vi "Populate_Do.vi"(8 "error in (no error)":errorcluster, 9 "Value":string, 10 "Lower case name":string, 11 "Copy Build Product Action in":refnum<class "Copy Build Product Action.lvclass">) -> (0 "error out":errorcluster, 1 "Success?":bool, 3 "Copy Build Product Action out":refnum<class "Copy Build Product Action.lvclass">)   [LabVIEW 2020, in "ProjectBuilder.lvlib" / "Copy Build Product Action.lvclass"]
uses:
  Copy Build Product Action.lvclass
  Copy Build Product Action.lvclass/Copy Build Product Action.ctl
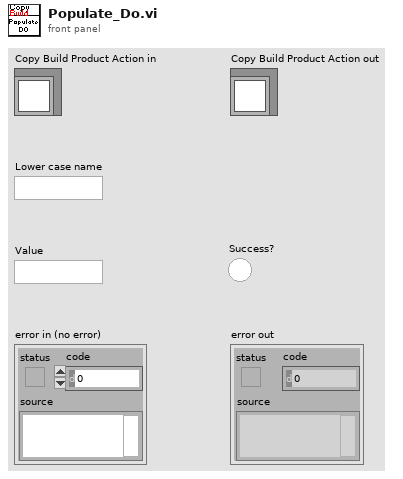
[diagram p1: front panel]
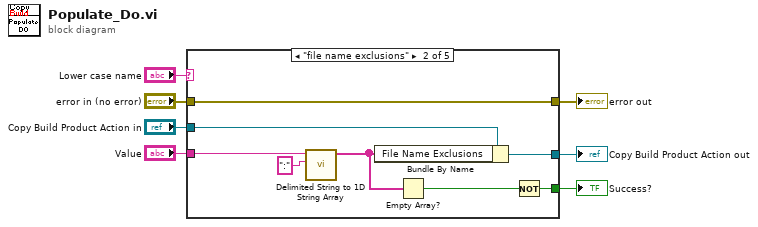
[diagram p0: block diagram]
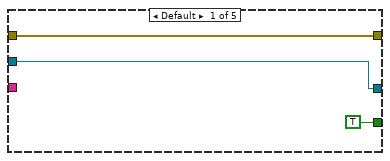
[diagram p2: hidden frame]
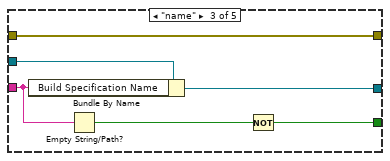
[diagram p3: hidden frame]
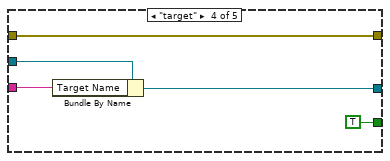
[diagram p4: hidden frame]
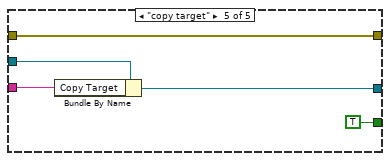
[diagram p5: hidden frame]
diagram:
  n1 = case shown="\"file name exclusions\"" "Lower case name" {
    tunnel: [TRUE w15 w20 TRUE TRUE] -> w6
    tunnel: [w9 w12 w23 w28 w33] -> w3
    tunnel: "Copy Build Product Action in" -> [w9 w14 w24 w29 w34]
    tunnel: [w8 w11 w19 w26 w31] -> w1
    tunnel: "error in (no error)" -> [w8 w11 w19 w26 w31]
    tunnel: "Value" -> [_ w18 w22 w27 w32]
    frame Default {
    }
    frame "file name exclusions" {
      n2 = call <vilib>:"Delimited String to 1D String Array.vi"("delimiter"=":", "delimited string"=w18) -> ("string array"=w13:string[])  [unwired: 9 in]
      n3 = Bundle By Name(cluster=w14, "File Name Exclusions"=w13) -> (w12:refnum<class "Copy Build Product Action.lvclass">)
      n4 = Empty Array?(array=w13) -> (empty?=w16:bool)
      n5 = Not(x=w16) -> (.not. x?=w15:bool)
    }
    frame "name" {
      n6 = Bundle By Name(cluster=w24, "Build Specification Name"=w22) -> (w23:refnum<class "Copy Build Product Action.lvclass">)
      n7 = Empty String/Path?(string/path=w22) -> (empty?=w21:bool)
      n8 = Not(x=w21) -> (.not. x?=w20:bool)
    }
    frame "target" {
      n9 = Bundle By Name(cluster=w29, "Target Name"=w27) -> (w28:refnum<class "Copy Build Product Action.lvclass">)
    }
    frame "copy target" {
      n10 = Bundle By Name(cluster=w34, "Copy Target"=w32) -> (w33:refnum<class "Copy Build Product Action.lvclass">)
    }
  }
  "error out" <- w1
  "Copy Build Product Action out" <- w3
  "Success?" <- w6
